vi "timing data doubles.vi"() -> ()   [LabVIEW 2009]
uses:
  <vilib>/Utility/file.llb/Write To Spreadsheet File (DBL).vi
  <vilib>/Utility/file.llb/Read From Spreadsheet File (DBL).vi
panel:
  in  "Path 2":path
  out "appended array":dbl[][](array[numeric])
  out "points":dbl[](array[numeric])
  out "ser":dbl[](array[numeric])
  out "frames":i32[](array[numeric])
  out "points":i32[](array[numeric])
  out "service":i32[](array[numeric])
  out "array w/ subset deleted":dbl[][](array[numeric])
  in  "Path":path
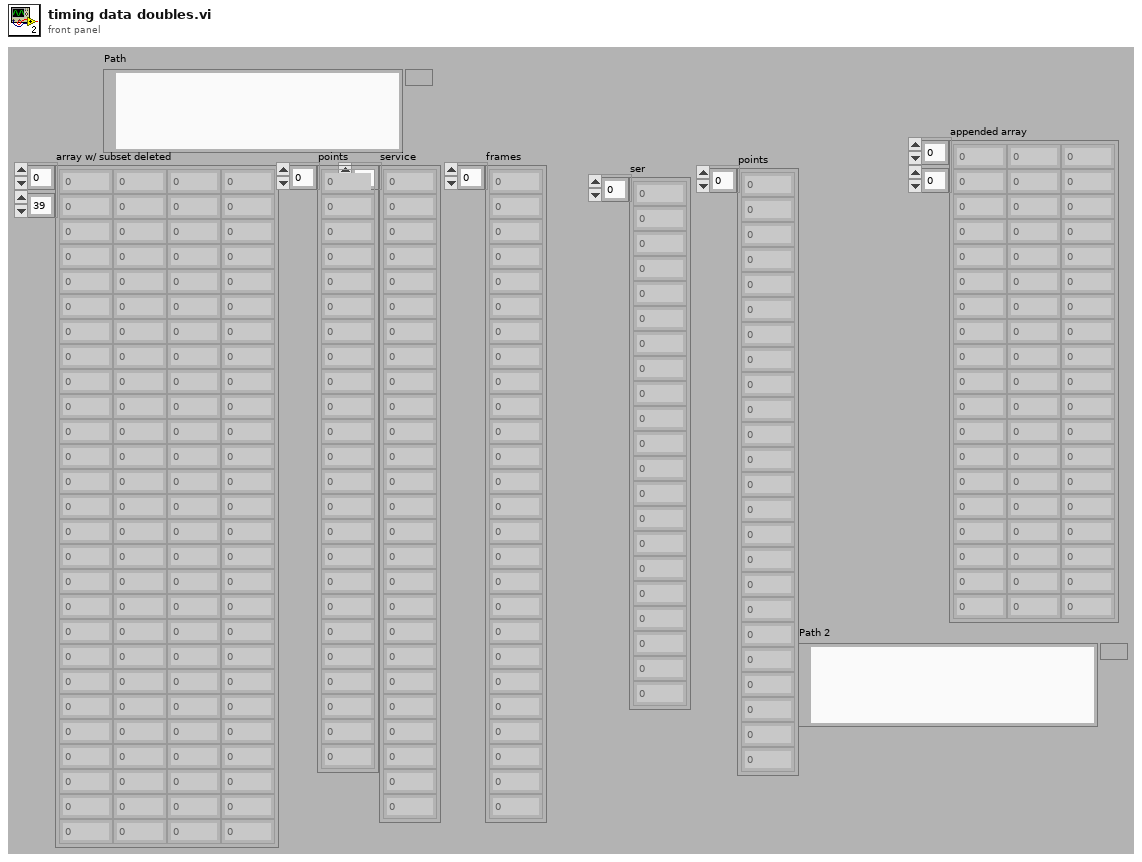
[diagram p1: front panel]
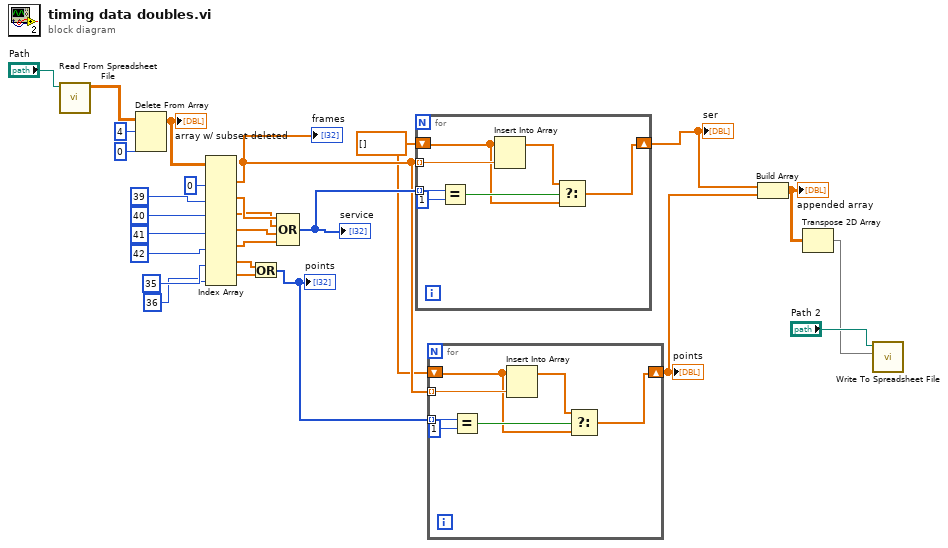
[diagram p0: block diagram]
diagram:
  w6 = dbl[] []
  n1 = call-poly <vilib>:"Read From Spreadsheet File.vi"("file path (dialog if empty)"="Path") -> ("all rows"=w26:dbl[][])  [unwired: 6 in, 4 out]
  n2 = Delete From Array(array=w26, length=4, index (row)=0) -> (array with subset deleted=w10:dbl[][])  [unwired: 1 in, 1 out]
  "array w/ subset deleted" <- w10
  n3 = Index Array(array=w10, index (col) #1=0 ("disabled index (col)"), index (col) #2=39 ("index (col)"), index (col) #3=40 ("disabled index (col)"), index (col) #4=41 ("index (col)"), index (col) #5=42 ("disabled index (col)"), index (col) #6=35 ("index (col)"), index (col) #7=36 ("disabled index (col)")) -> (element #1=w7:dbl[], element #2=w16:dbl[], element #3=w15:dbl[], element #4=w14:dbl[], element #5=w13:dbl[], element #6=w12:dbl[], element #7=w11:dbl[])  [unwired: 7 in]
  "frames" <- w7
  n4 = Or(x=w12, y=w11) -> (x .or. y?=w8:i32[])
  "points" <- w8
  n5 = Compound Arithmetic op=OR(w16, w15, w14, w13) -> (w9:i32[])
  "service" <- w9
  n6 = for {
    tunnel: w7 -> [w31] mode=indexing
    tunnel: w9 -> [w34] mode=indexing
    shift-right: [w30] -> w5
    shift-left: w6 -> [w28]
    n7 = Equal?(x=w34, y=1) -> (x = y?=w32:bool)
    n8 = Insert Into Array(array=w28, new element=w31) -> (w29:dbl[])  [unwired: 1 in]
    n9 = Select(t=w29, s=w32, f=w28) -> (s? t:f=w30:dbl[])
  }
  "ser" <- w5
  n10 = for {
    tunnel: w7 -> [w38] mode=indexing
    tunnel: w8 -> [w41] mode=indexing
    shift-right: [w37] -> w4
    shift-left: w6 -> [w35]
    n11 = Equal?(x=w41, y=1) -> (x = y?=w39:bool)
    n12 = Insert Into Array(array=w35, new element=w38) -> (w36:dbl[])  [unwired: 1 in]
    n13 = Select(t=w36, s=w39, f=w35) -> (s? t:f=w37:dbl[])
  }
  "points" <- w4
  n14 = Build Array(w5, w4) -> (w3:dbl[][])
  "appended array" <- w3
  n15 = Transpose 2D Array(2D array=w3) -> (transposed array=w1:dbl[][])
  n16 = call-poly <vilib>:"Write To Spreadsheet File.vi"("2D data"=w1, "file path (dialog if empty)"="Path 2") -> ()  [unwired: 6 in, 1 out]
